vi "Create String for Cluster in Result.vi"(0 "VI Reference":refnum<vi>, 2 "Output CLuster[]":string[](array[string]), 5 "Ctl Refnum":refnum<vi>, 7 "Result Cluster":refnum<vi>, 11 "error in (no error)":errorcluster) -> (4 "Output Clusters":string[](array[string]), 15 "error out":errorcluster)   [LabVIEW 2021, in "Converter.lvlib"]
uses:
  Conversion Logic/Converter.lvlib
  <vilib>/Utility/miscctls.llb/LVPositionTypeDef.ctl
  Converter Reusables.lvlib
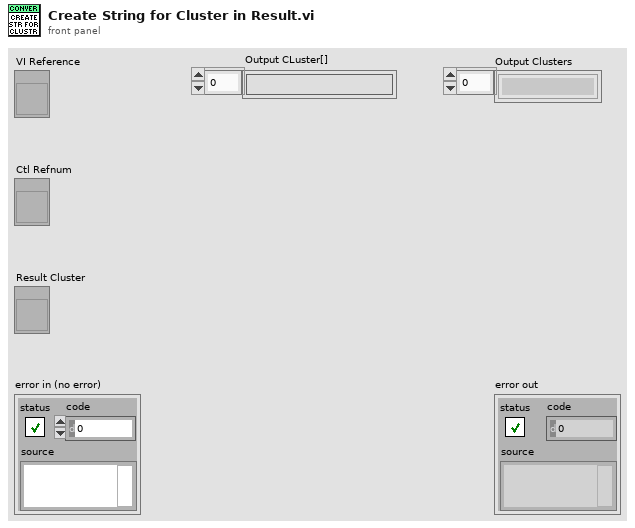
[diagram p1: front panel]
types:
  T1 = typedef "LVPositionTypeDef.ctl" = cluster{"Left":i32, "Top":i32}
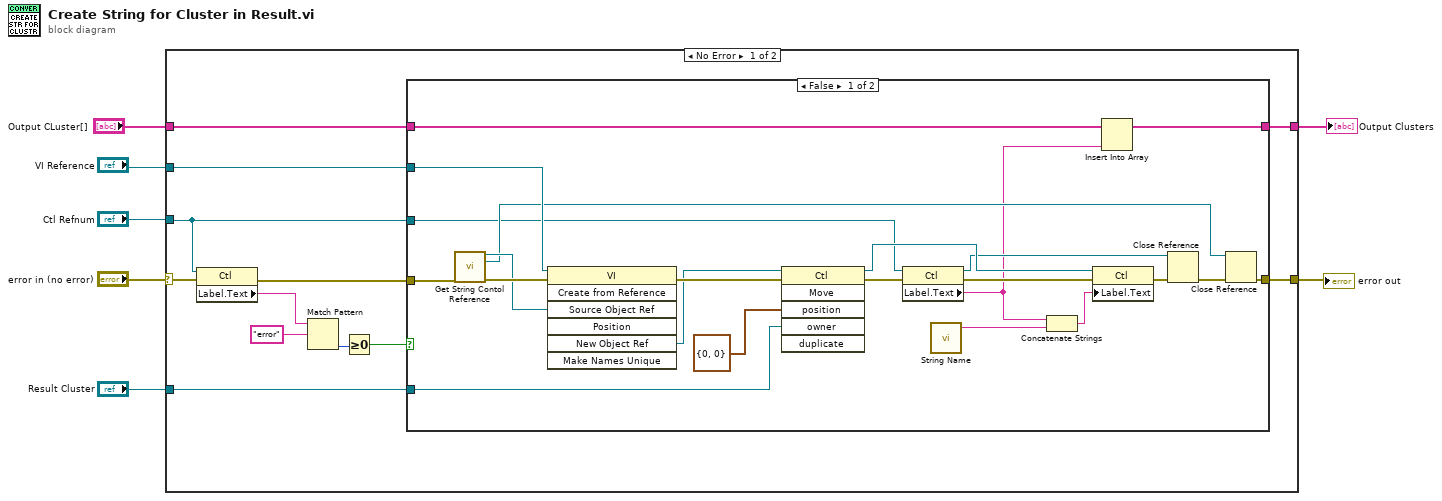
[diagram p0: block diagram]
diagram:
  n1 = case shown="No Error" "error in (no error)" {
    selector: "error in (no error)" -> [w15 w45]
    tunnel: [w17 w45] -> w7
    tunnel: "VI Reference" -> [w19 _]
    tunnel: "Result Cluster" -> [w18 _]
    tunnel: "Ctl Refnum" -> [w16 _]
    tunnel: "Output CLuster[]" -> [w9 w44]
    tunnel: [w8 w44] -> w1
    frame No Error {
      n2 = property class="Ctl"(reference=w16, error in=w15) -> (error out=w14:errorcluster, "Label.Text"=w11:string)  [unwired: 1 out]
      n3 = Match Pattern(string=w11, regular expression="error") -> (offset past match=w12:i32)  [unwired: 1 in, 3 out]
      n4 = Greater Or Equal To 0?(x=w12) -> (x >= 0?=w10:bool)
      n5 = case shown="False" w10 {
        tunnel: w19 -> [w40 _]
        tunnel: w18 -> [w39 _]
        tunnel: [w27 w42] -> w17
        tunnel: w16 -> [w24 _]
        tunnel: w14 -> [w23 w42]
        tunnel: w9 -> [w21 w43]
        tunnel: [w20 w43] -> w8
        frame False {
          n6 = call "Get String Contol Reference.vi"("error in (no error)"=w23) -> ("String"=w36:refnum<vi>, "vi reference"=w26:refnum<vi>, "error out"=w41:errorcluster)  [unwired: 12 in]
          n7 = invoke class="VI" method="Create from Reference"(reference=w40, error in=w41, "Source Object Ref"=w36) -> (error out=w38:errorcluster, "New Object Ref"=w37:refnum<vi>)  [unwired: 4 in, 5 out]
          n8 = invoke class="Ctl" method="Move"(reference=w37, error in=w38, "position"=T1 {"Left"=0, "Top"=0}, "owner"=w39) -> (reference out=w31:refnum<vi>, error out=w35:errorcluster)  [unwired: 2 in, 4 out]
          n9 = property class="Ctl"(reference=w24, error in=w35) -> (reference out=w29:refnum<vi>, error out=w32:errorcluster, "Label.Text"=w22:string)
          n10 = call "String Name.vi"() -> ("Postfix"=w34:string)  [unwired: 15 in]
          n11 = Concatenate Strings(w22, w34) -> (w33:string)
          n12 = property class="Ctl"(reference=w31, error in=w32, "Label.Text"=w33) -> (error out=w30:errorcluster)  [unwired: 1 out]
          n13 = Insert Into Array(array=w21, new element=w22) -> (w20:string[])  [unwired: 1 in]
          n14 = Close Reference(reference=w29, error in (no error)=w30) -> (error out=w28:errorcluster)
          n15 = Close Reference(reference=w26, error in (no error)=w28) -> (error out=w27:errorcluster)
        }
        frame True {
        }
      }
    }
    frame Error {
    }
  }
  "error out" <- w7
  "Output Clusters" <- w1
